vi "MOCKBEAR_Pull_Sample.vi"(0 "MOCKBEAR in":refnum<class "MOCKBEAR.lvclass">, 1 "FEA Model":refnum<class "FEA_Model.lvclass">, 5 "error in (no error)":errorcluster) -> (14 "Accelerometer sample":dbl[](array[numeric]), 15 "Last pin pos node":i32, 16 "Sample Time":u32, 17 "Last pin pos meter":dbl, 18 "looping":bool, 19 "error out":errorcluster)   [LabVIEW 2021, in "MOCKBEAR.lvclass"]
uses:
  MOCKBEAR.lvclass
  FEA_Model/FEA_Model.lvclass
  MOCKBEAR.lvclass/MOCKBEAR.ctl
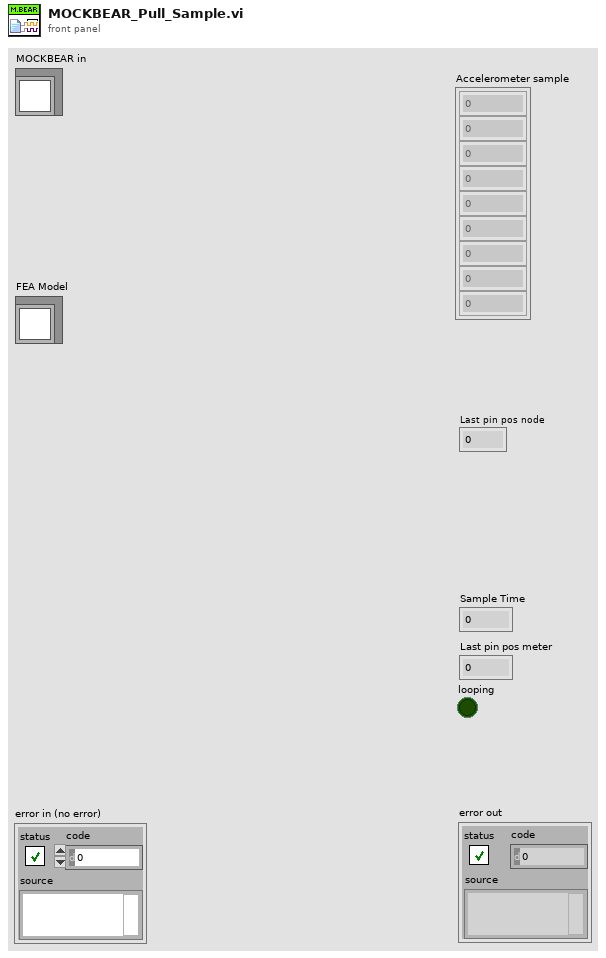
[diagram p1: front panel]
types:
  T1 = enum16{"Scalar Particle to Meter", "Scalar Node to Meter", "Scalar Meter to Particle", "Scalar Meter to Node", "Array Particle to Meter", "Array Node to Meter", "Array Meter to Particle", "Array Meter to Node"}
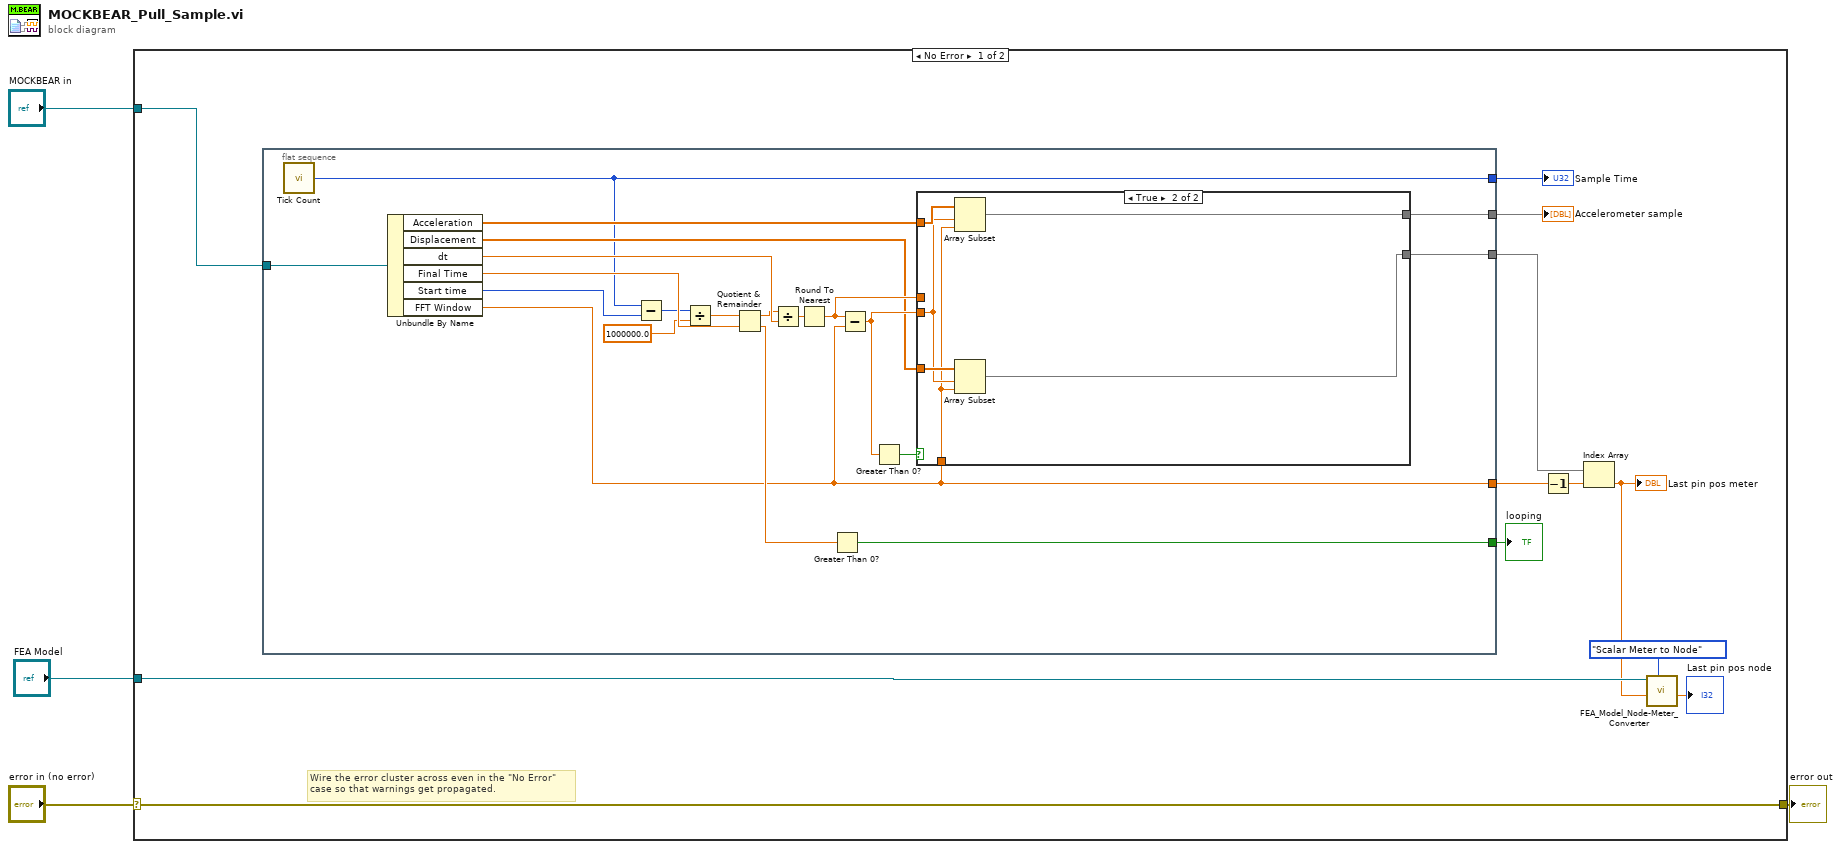
[diagram p0: block diagram]
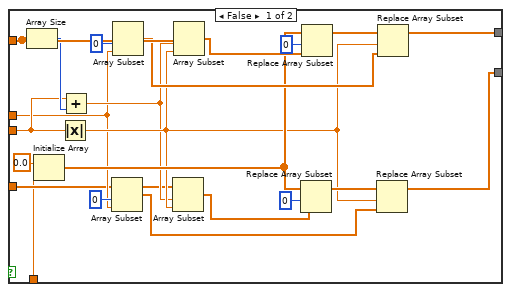
[diagram p2: hidden frame]
diagram:
  n1 = case shown="No Error" "error in (no error)" {
    selector: "error in (no error)" -> [w16 w65]
    tunnel: [w16 w65] -> w3
    tunnel: "MOCKBEAR in" -> [w9 _]
    tunnel: "FEA Model" -> [w8 _]
    frame No Error {
      # "Wire the error cluster across even in the \"No Error\"\ncase so that warnings get propagated."
      n2 = flat-sequence {
        tunnel: w9 -> [w36]
        tunnel: [w33] -> w15
        tunnel: [w29] -> w11
        tunnel: [w24] -> w14
        tunnel: [w17] -> w12
        tunnel: [w22] -> w10
        frame #0 {
          n3 = call "Tick Count"() -> ("Tick Count(uSec)"=w24:u32)
          n4 = Unbundle By Name(w36) -> ("Acceleration"=w34:dbl[], "Displacement"=w26:dbl[], "dt"=w27:dbl, "Final Time"=w28:dbl, "Start time"=w25:u32, "FFT Window"=w17:dbl)
          n5 = Subtract(x=w24, y=w25) -> (x-y=w19:u32)
          n6 = Divide(x=w19, y=1000000.0) -> (x/y=w20:dbl)
          n7 = Quotient & Remainder(x=w20, y=w28) -> (x-y*floor(x/y)=w23:dbl, floor(x/y)=w21:dbl)
          n8 = Divide(x=w23, y=w27) -> (x/y=w35:dbl)
          n9 = Round To Nearest(number=w35) -> (nearest integer value=w30:dbl)
          n10 = Greater Than 0?(x=w21) -> (x > 0?=w22:bool)
          n11 = Subtract(x=w30, y=w17) -> (x-y=w31:dbl)
          n12 = Greater Than 0?(x=w31) -> (x > 0?=w32:bool)
          n13 = case shown="True" w32 {
            tunnel: w31 -> [w50 w61]
            tunnel: w34 -> [w58 w64]
            tunnel: [w53 w63] -> w33
            tunnel: w30 -> [w41 _]
            tunnel: [w49 w60] -> w29
            tunnel: w26 -> [w40 w62]
            tunnel: w17 -> [w37 w59]
            frame False {
              n14 = Array Size(array=w58) -> (size(s)=w57:i32)
              n15 = Initialize Array(0.0 ("element"), w37) -> (w47:dbl[])
              n16 = Absolute Value(x=w50) -> (abs(x)=w44:dbl)
              n17 = Add(x=w50, y=w57) -> (x+y=w43:dbl)
              n18 = Array Subset(array=w40, index=0, length=w41) -> (w39:dbl[])
              n19 = Array Subset(array=w58, index=0, length=w41) -> (w48:dbl[])
              n20 = Array Subset(array=w40, index=w43, length=w44) -> (w38:dbl[])
              n21 = Array Subset(array=w58, index=w43, length=w44) -> (w52:dbl[])
              n22 = Replace Array Subset(array=w47, new element=w38, index=0) -> (w46:dbl[])
              n23 = Replace Array Subset(array=w47, new element=w52, index=0) -> (w54:dbl[])
              n24 = Replace Array Subset(array=w46, new element=w39, index=w44) -> (w49:dbl[])
              n25 = Replace Array Subset(array=w54, new element=w48, index=w44) -> (w53:dbl[])
            }
            frame True {
              n26 = Array Subset(array=w64, index=w61, length=w59) -> (w63:dbl[])
              n27 = Array Subset(array=w62, index=w61, length=w59) -> (w60:dbl[])
            }
          }
        }
      }
      n28 = Decrement(x=w12) -> (x-1=w13:dbl)
      n29 = Index Array(array=w11, index=w13) -> (element=w7:dbl)
      "Last pin pos meter" <- w7
      n30 = call "FEA_Model_Node-Meter_Converter.vi"("Conversion Mode"=T1."Scalar Meter to Node", "Scalar in"=w7, "FEA_Model in"=w8) -> ("Scalar out"=→"Last pin pos node":dbl)  [unwired: 5 in, 3 out]
      "Accelerometer sample" <- w15
      "Sample Time" <- w14
      "looping" <- w10
    }
    frame Error {
    }
  }
  "error out" <- w3
